vi "Read File Preamble.vi"(11 "file preamble":string) -> (0 "vertical range":dbl, 1 "sample rate":dbl, 2 "center frequency":dbl, 3 "time":string)   [LabVIEW 2018]
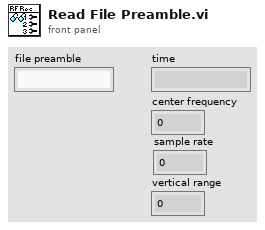
[diagram p1: front panel]
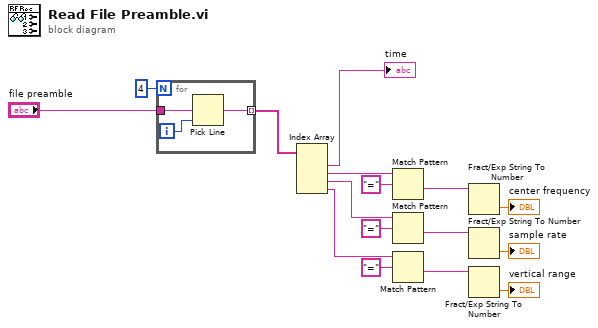
[diagram p0: block diagram]
diagram:
  n1 = for {
    N: 4 -> [_]
    tunnel: [w19] -> w10 mode=indexing
    tunnel: "file preamble" -> [w17]
    i -> [w18]
    n2 = Pick Line(multi-line string=w17, line index=w18) -> (output string=w19:string)  [unwired: 1 in]
  }
  n3 = Index Array(array=w10) -> (element #1=→"time":string, element #2=w11:string, element #3=w14:string, element #4=w16:string)  [unwired: 4 in]
  n4 = Match Pattern(string=w11, regular expression="=" ("search string/char (-)")) -> (after substring=w6:string)  [unwired: 1 in, 3 out]
  n5 = Match Pattern(string=w14, regular expression="=" ("search string/char (-)")) -> (after substring=w5:string)  [unwired: 1 in, 3 out]
  n6 = Match Pattern(string=w16, regular expression="=" ("search string/char (-)")) -> (after substring=w4:string)  [unwired: 1 in, 3 out]
  n7 = Fract/Exp String To Number(string=w6) -> (number=→"center frequency":dbl)  [unwired: 3 in, 1 out]
  n8 = Fract/Exp String To Number(string=w5) -> (number=→"sample rate":dbl)  [unwired: 3 in, 1 out]
  n9 = Fract/Exp String To Number(string=w4) -> (number=→"vertical range":dbl)  [unwired: 3 in, 1 out]
